vi "Upper Target Loop.vi"(11 "Camera Name":string="cam0") -> ()   [LabVIEW 2025]
uses:
  <vilib>/vision/NI_Vision_Development_Module.lvlib
  <vilib>/vision/Image Controls.llb/IMAQ Image.ctl
  <vilib>/Utility/config.llb/NI_LVConfig.lvlib
  <vilib>/Utility/config.llb/Write Key (String).vi
  Camera Set Up/Event/Event Setup Types.ctl
  <vilib>/Analysis/NI_AALBase.lvlib
  <vilib>/Analysis/baseanly.llb/Mean (DBL).vi
  <vilib>/Rock Robotics/Network Tables/NT Write Number.vi
  <vilib>/Utility/config.llb/Read Key (String).vi
  Camera Set Up/Ctrl/Camera Setup Cluster.ctl
panel:
  in  "Main":enum32{"Page 1", "Page 2"}(tab)
  in  "Settings":bool
  in  "Save":bool
  in  "Tools":bool
  out "Angle Array":dbl[](array[numeric]) format="%.1f"
  out "Distance  Array":dbl[](array[numeric]) format="%.1f"
  out "Avg Angle":dbl format="%0.2f"
  out "Avg Distance":dbl format="%0.2f"
  out "Image":T1(plugin-control)
  in  "Home":bool
  out "Mask":T1(plugin-control)
  in  "Dilate":bool
  in  "Color Range":T2={"Hue"={21.620689392089844, 69.62068939208984}, "Sat"={66.41378784179688, 255.0}, "Val"={96.0, 255.0}} {"Hue" scale=0.0..255.0 scale format="%#_3g"}
  in  "Height to center of target \n from floor (hp (in))":dbl=104.0 format="%#_13g"
  in  "FOV":dbl=120.0
  in  "Robot Calibration":T3={"Camera Height on robot (in)"=26.7, "Camera Angle on the robot (deg)"=21.6, "Slope"=0.946, "Offset"=10.775} {"Offset" format="%#_13g"; "Slope" format="%#_13g"; "Camera Angle on the robot (deg)" format="%#_13g"; "Camera Height on robot (in)" format="%#_13g"}
  in  "Score Threshold %":dbl=70.0
  in  "Size Limit %":dbl=0.02 format="%#_13g"
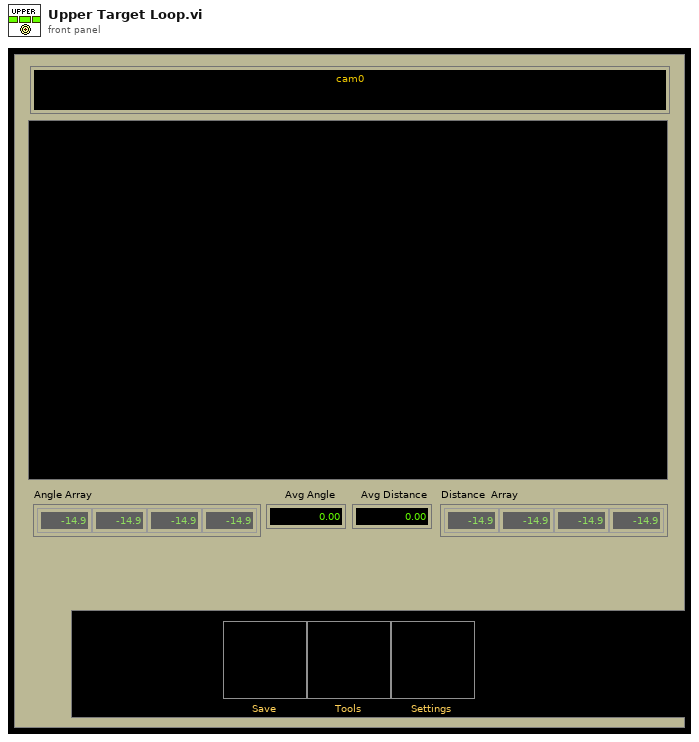
[diagram p1: front panel]
types:
  T1 = typedef "IMAQ Image.ctl" = refnum<image>
  T2 = cluster{"Hue":cluster{dbl, dbl}, "Sat":cluster{dbl, dbl}, "Val":cluster{dbl, dbl}}
  T3 = typedef "Camera Setup Cluster.ctl" = cluster{"Camera Height on robot (in)":dbl, "Camera Angle on the robot (deg)":dbl, "Slope":dbl, "Offset":dbl}
  T4 = typedef "Image Type" = u32
  T5 = typedef "Particle Parameters" = i32
  T6 = enum32{"AutoM", "Close", "Dilate", "Erode", "Gradient", "Gradient out", "Gradient in", "Hit miss", "Open", "PClose", "POpen", "Thick", "Thin"}
  T7 = typedef "Event Setup Types.ctl" = enum16{"Default", "Camera Loop Started", "GreyScale", "Reset Camera Settings", "Reset Team Number", "Save Data", "Setting Changed", "Update Video Mode", "Video Mode Changed", "Exit"}
  T8 = typedef "Event Setup Types.ctl" = enum16{"Default", "Camera Loop Started", "Close Settings", "GreyScale", "Open Front Panel", "Reset Team Number", "Save Data", "Exit"}
  T9 = typedef "Target Fields.ctl" = cluster{"diameter points":cluster{"first point":cluster{"x":dbl, "y":dbl}, "projected point":cluster{"x":dbl, "y":dbl}}, "normalized center":cluster{"x":dbl, "y":dbl}, "Overall Score":dbl, "Area Score":dbl, "Moment Score":dbl, "Aspect Score":dbl, "Distance (ft)":dbl, "Upper Goal":bool}
  T10 = typedef "NI_LVConfig.lvlib/Config Data RefNum.ctl" = refnum<k1>
  T11 = cluster{cluster{"Lower":dbl, "Upper":dbl}, cluster{"Lower":dbl, "Upper":dbl}, cluster{"Lower":dbl, "Upper":dbl}}
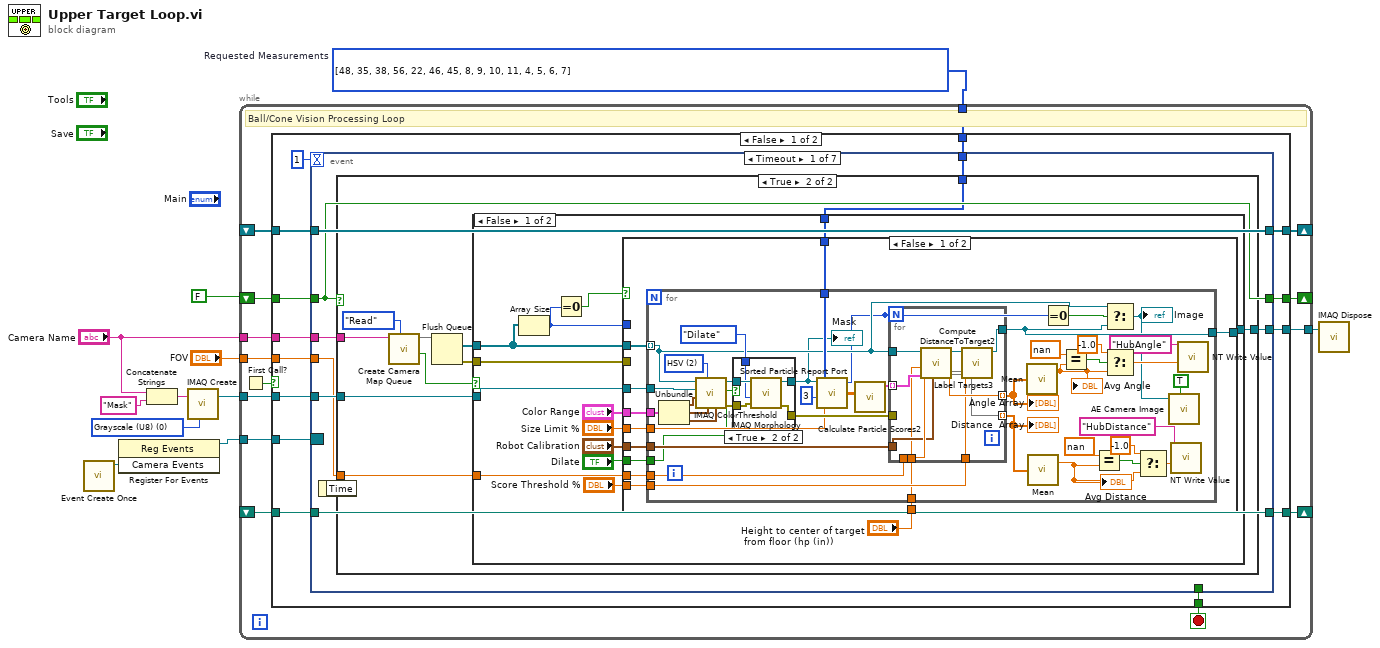
[diagram p0: block diagram]
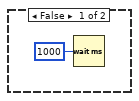
[diagram p2: hidden frame]
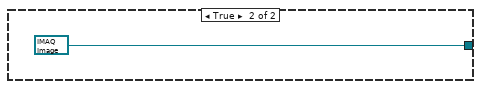
[diagram p4: hidden frame]
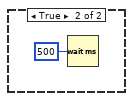
[diagram p5: hidden frame]
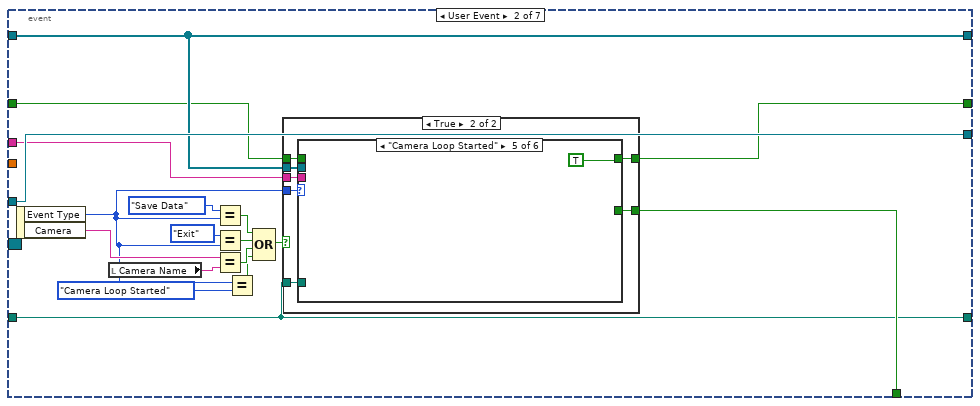
[diagram p6: hidden frame]
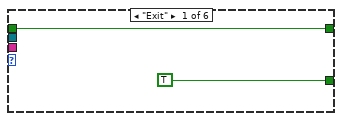
[diagram p8: hidden frame]
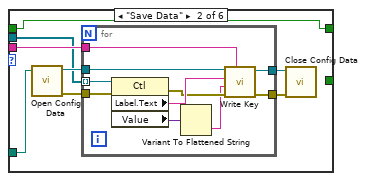
[diagram p9: hidden frame]
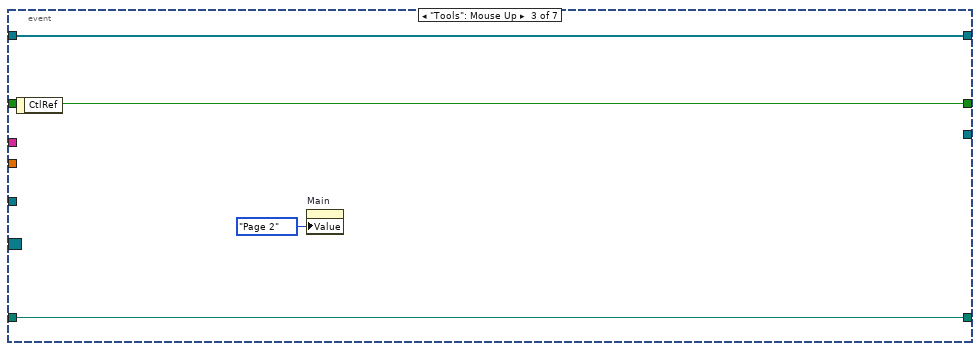
[diagram p13: hidden frame]
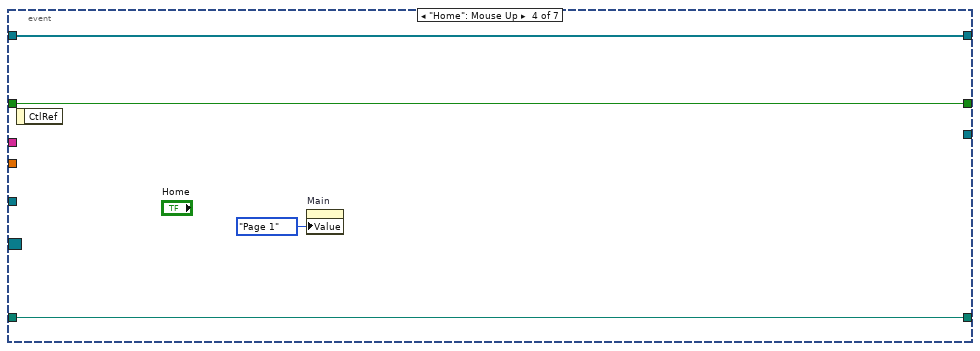
[diagram p14: hidden frame]
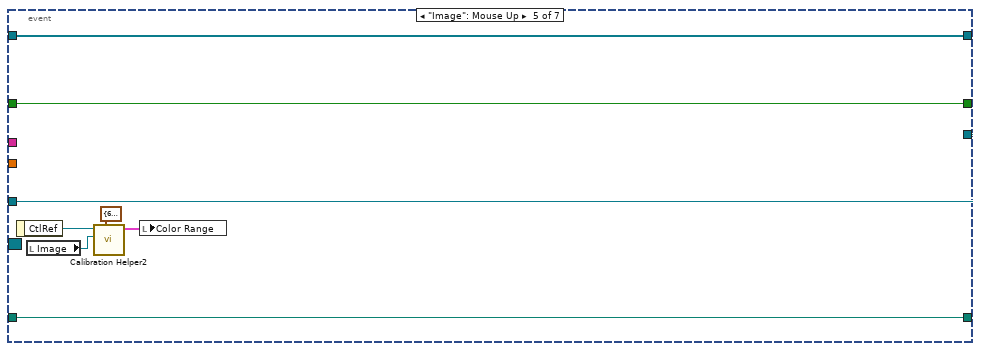
[diagram p15: hidden frame]
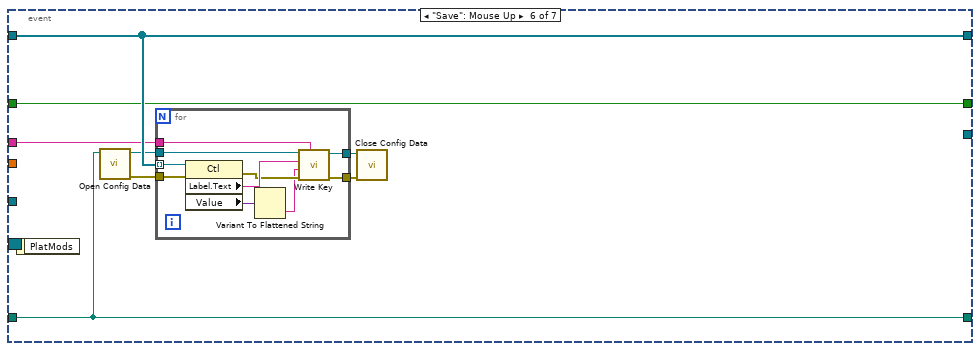
[diagram p16: hidden frame]
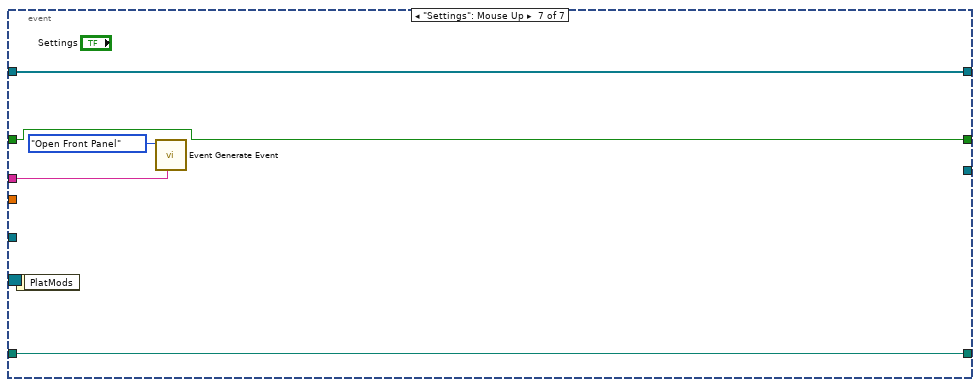
[diagram p17: hidden frame]
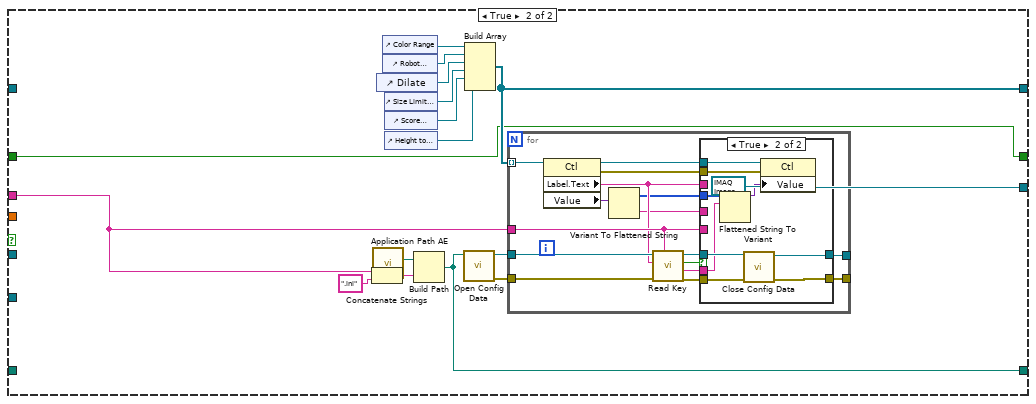
[diagram p18: hidden frame]
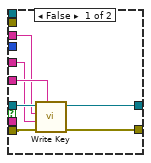
[diagram p19: hidden frame]
diagram:
  w7 = T4 0 items=["Grayscale (U8)", "Grayscale (I16)", "Grayscale (SGL)", "Complex (CSG)", "RGB (U32)", "HSL (U32)", "RGB (U64)", "Grayscale (U16)"] ("Image Type")
  w4 = T5[] [48, 35, 38, 56, 22, 46, 45, 8, 9, 10, 11, 4, 5, 6, 7] items=["Center of Mass X", "Center of Mass Y", "First Pixel X", "First Pixel Y", "Bounding Rect Left", "Bounding Rect Top", "Bounding Rect Right", "Bounding Rect Bottom", "Max Feret Diameter Start X", "Max Feret Diameter Start Y", "Max Feret Diameter End X", "Max Feret Diameter End Y", "Max Horiz. Segment Length Left", "Max Horiz. Segment Length Right", "Max Horiz. Segment Length Row", "-", "Bounding Rect Width", "Bounding Rect Height", "Bounding Rect Diagonal", "Perimeter", "Convex Hull Perimeter", "Holes' Perimeter", "Max Feret Diameter", "Equivalent Ellipse Major Axis", "Equivalent Ellipse Minor Axis", "Equivalent Ellipse Minor Axis (Feret)", "Equivalent Rect Long Side", "Equivalent Rect Short Side", "Equivalent Rect Diagonal", "Equivalent Rect Short Side (Feret)", "Average Horiz. Segment Length", "Average Vert. Segment Length", "Hydraulic Radius", "Waddel Disk Diameter", "-", "Area", "Holes' Area", "Particle & Holes' Area", "Convex Hull Area", "Image Area", "-", "Number of Holes", "Number of Horiz. Segments", "Number of Vert. Segments", "-", "Orientation", "Max Feret Diameter Orientation", "-", "% Area/Image Area", "% Area/(Particle & Holes' Area)", "Ratio of Equivalent Ellipse Axes", "Ratio of Equivalent Rect Sides", "-", "Elongation Factor", "Compactness Factor", "Heywood Circularity Factor", "Type Factor", "-", "Sum X", "Sum Y", "Sum XX", "Sum XY", "Sum YY", "Sum XXX", "Sum XXY", "Sum XYY", "Sum YYY", "-", "Moment of Inertia XX", "Moment of Inertia XY", "Moment of Inertia YY", "Moment of Inertia XXX", "Moment of Inertia XXY", "Moment of Inertia XYY", "Moment of Inertia YYY", "Norm. Moment of Inertia XX", "Norm. Moment of Inertia XY", "Norm. Moment of Inertia YY", "Norm. Moment of Inertia XXX", "Norm. Moment of Inertia XXY", "Norm. Moment of Inertia XYY", "Norm. Moment of Inertia YYY", "Hu Moment 1", "Hu Moment 2", "Hu Moment 3", "Hu Moment 4", "Hu Moment 5", "Hu Moment 6", "Hu Moment 7"]  # Requested Measurements
  n1 = call "Event Create Once.vi"() -> ("Camera Events"=w9:refnum<user-event>)  [unwired: 10 in, 1 out]
  n2 = register-events(w9) -> (reference out=w8:refnum<event-registration>)  [unwired: 2 in, 1 out]
  n3 = Concatenate Strings("Camera Name", "Mask" ("string")) -> (w6:string)
  n4 = call "IMAQ Create"("Image Name"=w6, "Image Type"=w7) -> ("New Image"=w11:T1)  [unwired: 2 in, 2 out]
  n5 = while {
    tunnel: w11 -> [w25]
    tunnel: w4 -> [w24]
    tunnel: [w23] -> w10
    tunnel: w8 -> [w22]
    tunnel: "FOV" -> [w20]
    tunnel: "Camera Name" -> [w19]
    shift-right: [w17] -> _
    shift-left: _ -> [w16]
    shift-right: [w15] -> _
    shift-left: _ -> [w14]
    shift-right: [w12] -> _
    shift-left: FALSE -> [w13]
    stop <- w21 stop-if-true
    # "Ball/Cone Vision Processing Loop"
    n6 = First Call?() -> (First Call?: T/F=w18:bool)
    n7 = case shown="False" w18 {
      tunnel: w25 -> [w39 _]
      tunnel: w24 -> [w38 _]
      tunnel: [w37 T1 refnum ("New Image")] -> w23
      tunnel: w22 -> [w35 _]
      tunnel: [w34 _] -> w21
      tunnel: w20 -> [w33 _]
      tunnel: w19 -> [w32 w245]
      tunnel: [w30 w244] -> w17
      tunnel: w16 -> [w31 _]
      tunnel: [w28 w243] -> w15
      tunnel: w14 -> [w29 _]
      tunnel: w13 -> [w27 w234]
      tunnel: [w26 w234] -> w12
      frame False {
        n8 = event shown="[0] Timeout" {
          selector: w35 -> [_ _ _ _ _ _ _]
          dyn-events: _ -> [_ _ _ _ _ _ _]
          timeout: 1 -> [_ _ _ _ _ _ _]
          tunnel: w39 -> [w45 w162 _ _ w208 _ _]
          tunnel: w38 -> [w43 _ _ _ _ _ _]
          tunnel: [w42 w162 _ _ w208 _ _] -> w37
          tunnel: [_ w161 _ _ _ _ _] -> w34
          tunnel: w33 -> [w44 _ _ _ _ _ _]
          tunnel: w32 -> [w41 w160 _ _ _ w216 w230]
          tunnel: w31 -> [w47 w158 w198 w202 w207 w217 w233]
          tunnel: [w47 w158 w198 w202 w207 w217 w233] -> w30
          tunnel: w29 -> [w46 w159 w197 w201 w206 w218 w232]
          tunnel: [w46 w159 w197 w201 w206 w218 w232] -> w28
          tunnel: [w40 w148 w195 w199 w203 w211 w229] -> w26
          tunnel: w27 -> [w40 w149 w195 w199 w203 w211 w229]
          event Timeout {
            n9 = event-data() -> ()  [unwired: 1 in, 1 out]
            n10 = case shown="True" w40 {
              tunnel: w45 -> [_ w57]
              tunnel: w44 -> [_ w56]
              tunnel: w43 -> [_ w55]
              tunnel: [_ w54] -> w42
              tunnel: w41 -> [_ w50]
              frame False {
                n11 = Wait (ms)(milliseconds to wait=u32 1000) -> ()  [unwired: 1 out]
              }
              frame True {
                n12 = call "Create Camera Map Queue.vi"("Action"=enum16{"Read", "Write"}."Read", "Camera"=w50) -> ("key not found?"=w49:bool, 3:w53)  [unwired: 7 in, 1 out]
                n13 = Flush Queue(queue=w53) -> (remaining elements=w51:T1[], error out=w52:errorcluster)  [unwired: 1 in, 1 out]
                n14 = case shown="False" w49 {
                  tunnel: w57 -> [w70 _]
                  tunnel: w56 -> [w69 _]
                  tunnel: w55 -> [w68 _]
                  tunnel: [w66 _] -> w54
                  tunnel: w52 -> [w65 _]
                  tunnel: w51 -> [w63 _]
                  frame False {
                    n15 = Array Size(array=w63) -> (size(s)=w60:i32)
                    n16 = Equal To 0?(x=w60) -> (x = 0?=w59:bool)
                    n17 = case shown="False" w59 {
                      tunnel: w68 -> [w83 _]
                      tunnel: w70 -> [w82 _]
                      tunnel: [w77 T1 refnum ("Image out")] -> w66
                      tunnel: "Color Range" -> [w81 _]
                      tunnel: "Size Limit %" -> [w80 _]
                      tunnel: "Robot Calibration" -> [w79 _]
                      tunnel: w69 -> [w78 _]
                      tunnel: "Dilate" -> [w76 _]
                      tunnel: w63 -> [w75 _]
                      tunnel: w65 -> [_ _]
                      tunnel: "Score Threshold %" -> [w74 _]
                      tunnel: "Height to center of target \n from floor (hp (in))" -> [w73 _]
                      tunnel: w60 -> [_ _]
                      frame False {
                        n18 = for {
                          tunnel: w83 -> [w124]
                          tunnel: w82 -> [w120]
                          tunnel: [w116] -> w77
                          tunnel: w75 -> [w109] mode=indexing
                          tunnel: w81 -> [w108]
                          tunnel: w80 -> [w107]
                          tunnel: w79 -> [w106]
                          tunnel: w78 -> [w105]
                          tunnel: w76 -> [w103]
                          tunnel: w74 -> [w101]
                          tunnel: w73 -> [w96]
                          w114 = u16 2 items=["RGB", "HSL", "HSV", "HSI"] ("Color Mode")
                          n19 = Unbundle(w108) -> ("Hue"=w121:cluster{dbl, dbl}, "Sat"=w123:cluster{dbl, dbl}, "Val"=w122:cluster{dbl, dbl})
                          n20 = call "IMAQ ColorThreshold"("Blue or Luma or Val or Inten Range"=w122, "Green or Sat Range"=w123, "Color Mode"=w114, "Red or Hue Range"=w121, "Image Dst"=w120, "Image Src"=w109) -> ("error out"=w111:errorcluster, "Image Dst Out"=w113:T1)  [unwired: 4 in]
                          n21 = case shown="True" w103 {
                            tunnel: w113 -> [w126 w131]
                            tunnel: [w126 w130] -> w102
                            tunnel: T6."Dilate" ("Operation") -> [_ w129]
                            tunnel: w111 -> [w125 w128]
                            tunnel: [w125 w127] -> w110
                            frame False {
                            }
                            frame True {
                              n22 = call "IMAQ Morphology"("error in (no error)"=w128, "Operation"=w129, "Image Src"=w131) -> ("error out"=w127:errorcluster, "Image Dst Out"=w130:T1)  [unwired: 7 in]
                            }
                          }
                          "Mask" <- w102
                          n23 = call "Sorted Particle Report Port.vi"("Min Area Size %"=w107, "Particle Count Limit"=3 ("Particle Count"), "Pixel Measurements"=w124, "Image in"=w102) -> ("Sorted Data"=w118:dbl[][], "Particles"=w104:i32)  [unwired: 1 out]
                          n24 = call "Calculate Particle Scores2.vi"("Sorted Data"=w118) -> ("Scores"=w117:T9[])  [unwired: 10 in]
                          n25 = for {
                            N: w104 -> [_]
                            tunnel: w117 -> [w137] mode=indexing
                            tunnel: [w136] -> w97 mode=indexing
                            tunnel: w105 -> [w138]
                            tunnel: w106 -> [w135]
                            tunnel: w110 -> [_]
                            tunnel: w109 -> [w141]
                            tunnel: [w142] -> w116
                            tunnel: [w134] -> w100 mode=indexing
                            tunnel: w101 -> [w133]
                            tunnel: w96 -> [w132]
                            n26 = call "Compute DistanceToTarget2.vi"(6:w135, 8:w137, "Camera Type"=w132, "Line"=w138, "Image Src"=w141) -> (0:w139, "Distance (ft)"=w136:dbl, "Image Dst Out"=w140:T1, 4:w134)  [unwired: 3 in]
                            n27 = call "Label Targets3.vi"("Score Threshold"=w133, "results"=w139, "Image in"=w140) -> ("Image out"=w142:T1)  [unwired: 8 in]
                          }
                          "Angle Array" <- w97
                          "Distance  Array" <- w100
                          n28 = call-poly <vilib>:"Mean.vi"("X"=w97) -> ("mean"=w86:dbl)  [unwired: 1 out]
                          "Avg Angle" <- w86
                          n29 = call-poly <vilib>:"Mean.vi"("X"=w100) -> ("mean"=w92:dbl)  [unwired: 1 out]
                          "Avg Distance" <- w92
                          n30 = Equal To 0?(x=w104) -> (x = 0?=w115:bool)
                          n31 = Equal?(x=nan, y=w86) -> (x = y?=w89:bool)
                          n32 = Equal?(x=nan, y=w92) -> (x = y?=w94:bool)
                          n33 = Select(t=w109, s=w115, f=w116) -> (s? t:f=w85:T1)
                          "Image" <- w85
                          n34 = Select(t=-1.0, s=w89, f=w86) -> (s? t:f=w87:dbl)
                          n35 = Select(t=-1.0, s=w94, f=w92) -> (s? t:f=w91:dbl)
                          n36 = call "AE Camera Image.vi"("Update"=TRUE, "Goal Camera"=w85) -> ()  [unwired: 9 in, 1 out]
                          n37 = call-poly <vilib>:"NT Write Value.vi"("value"=w91, "name"="HubDistance" ("Name")) -> ()  [unwired: 9 in, 1 out]
                          n38 = call-poly <vilib>:"NT Write Value.vi"("value"=w87, "name"="HubAngle" ("Name")) -> ()  [unwired: 9 in, 1 out]
                        }
                      }
                      frame True {
                      }
                    }
                  }
                  frame True {
                    n39 = Wait (ms)(milliseconds to wait=u32 500) -> ()  [unwired: 1 out]
                  }
                }
              }
            }
          }
          event User Event {
            n40 = event-data() -> ("Event Type"=w146:T7, "Camera"=w153:string)  [unwired: 1 in]
            n41 = local read "Camera Name"() -> (w152:string)
            n42 = Equal?(x=Event_Setup_Types."Save Data", y=w146) -> (x = y?=w154:bool)
            n43 = Equal?(x=Event_Setup_Types."Exit", y=w146) -> (x = y?=w156:bool)
            n44 = Equal?(x=w153, y=w152) -> (x = y?=w151:bool)
            n45 = Equal?(x=w146, y=Event_Setup_Types."Camera Loop Started" ("x")) -> (x = y?=w145:bool)
            n46 = Compound Arithmetic op=OR(w154, w156, w151, w145) -> (w150:bool)
            n47 = case shown="True" w150 {
              tunnel: w146 -> [_ w170]
              tunnel: [_ w169] -> w161
              tunnel: w160 -> [_ w168]
              tunnel: w159 -> [_ w167]
              tunnel: w158 -> [_ w166]
              tunnel: w149 -> [w163 w165]
              tunnel: [w163 w164] -> w148
              frame False {
              }
              frame True {
                n48 = case shown="\"Camera Loop Started\"" w170 {
                  tunnel: [TRUE _ _ _ _ _] -> w169
                  tunnel: w168 -> [_ w176 _ _ _ _]
                  tunnel: w167 -> [_ w175 _ _ _ _]
                  tunnel: w166 -> [_ w174 _ _ _ _]
                  tunnel: w165 -> [w171 w173 w191 w192 _ w194]
                  tunnel: [w171 w173 w191 w192 TRUE w194] -> w164
                  frame "Exit" {
                  }
                  frame "Save Data" {
                    n49 = call <vilib>:"Open Config Data.vi"("configuration file path"=w175) -> ("error out"=w177:errorcluster, "refnum"=w180:T10)  [unwired: 8 in, 1 out]
                    n50 = for {
                      tunnel: w174 -> [w188] mode=indexing
                      tunnel: w180 -> [w190]
                      tunnel: w176 -> [w189]
                      tunnel: [w185] -> w179
                      tunnel: [w183] -> w178
                      tunnel: w177 -> [w182]
                      n51 = property class="Ctl"(reference=w188, error in=w182) -> (error out=w184:errorcluster, "Label.Text"=w187:string, "Value"=w186:variant)  [unwired: 1 out]
                      n52 = Variant To Flattened String(Variant=w186) -> (data string=w181:string)  [unwired: 1 out]
                      n53 = call-poly <vilib>:"Write Key.vi"("section"=w189, "error in (no error)"=w184, "value"=w181, "key"=w187, "refnum"=w190) -> ("error out"=w183:errorcluster, "refnum out"=w185:T10)  [unwired: 4 in, 1 out]
                    }
                    n54 = call <vilib>:"Close Config Data.vi"("error in (no error)"=w178, "refnum"=w179) -> ()  [unwired: 8 in, 2 out]
                  }
                  frame Default {
                  }
                  frame "Default" {
                  }
                  frame "Camera Loop Started" {
                  }
                  frame "Default" {
                  }
                }
              }
            }
          }
          event "Tools": Mouse Up {
            n55 = event-data() -> ()  [unwired: 1 in, 1 out]
            n56 = property on="Main" class="TabCtl (strict)"("Value"=enum32{"Page 1", "Page 2"}."Page 2" ("Main")) -> ()  [unwired: 2 in, 2 out]
          }
          event "Home": Mouse Up {
            n57 = event-data() -> ()  [unwired: 1 in, 1 out]
            n58 = property on="Main" class="TabCtl (strict)"("Value"=enum32{"Page 1", "Page 2"}."Page 1" ("Main")) -> ()  [unwired: 2 in, 2 out]
          }
          event "Image": Mouse Up {
            n59 = event-data() -> ("CtlRef"=w205:refnum<vi>)  [unwired: 1 in]
            n60 = local read "Image"() -> (w204:T1)
            n61 = call "Calibration Helper2.vi"("Std Devs"=cluster{"H":dbl, "S":dbl, "V":dbl} {"H"=6.0, "S"=6.0, "V"=6.0} ("Std Devs Ball"), "Image"=w204, "Image Ctl Refnum"=w205) -> ("output color"=w209:T11)  [unwired: 7 in, 1 out]
            n62 = local write "Color Range"(w209) -> ()
          }
          event "Save": Mouse Up {
            n63 = event-data() -> ()  [unwired: 1 in, 1 out]
            n64 = call <vilib>:"Open Config Data.vi"("configuration file path"=w218) -> ("error out"=w212:errorcluster, "refnum"=w215:T10)  [unwired: 8 in, 1 out]
            n65 = for {
              tunnel: w217 -> [w226] mode=indexing
              tunnel: w215 -> [w228]
              tunnel: w216 -> [w227]
              tunnel: [w223] -> w214
              tunnel: [w221] -> w213
              tunnel: w212 -> [w220]
              n66 = property class="Ctl"(reference=w226, error in=w220) -> (error out=w222:errorcluster, "Label.Text"=w225:string, "Value"=w224:variant)  [unwired: 1 out]
              n67 = Variant To Flattened String(Variant=w224) -> (data string=w219:string)  [unwired: 1 out]
              n68 = call-poly <vilib>:"Write Key.vi"("section"=w227, "error in (no error)"=w222, "value"=w219, "key"=w225, "refnum"=w228) -> ("error out"=w221:errorcluster, "refnum out"=w223:T10)  [unwired: 4 in, 1 out]
            }
            n69 = call <vilib>:"Close Config Data.vi"("error in (no error)"=w213, "refnum"=w214) -> ()  [unwired: 8 in, 2 out]
          }
          event "Settings": Mouse Up {
            n70 = event-data() -> ()  [unwired: 1 in, 1 out]
            n71 = call "Event Generate Event.vi"("Camera Name"=w230, "Event Type"=Event_Setup_Types."Open Front Panel") -> ()  [unwired: 10 in]
          }
        }
      }
      frame True {
        n72 = Concatenate Strings(w245, ".ini" ("name or relative path")) -> (w250:string)
        n73 = call "Application Path AE.vi"() -> ("Application Path out"=w238:path)  [unwired: 11 in]
        n74 = control-ref of="Dilate"() -> (w239:refnum<vi>)
        n75 = control-ref of="Color Range"() -> (w241:refnum<vi>)
        n76 = control-ref of="Robot Calibration"() -> (w240:refnum<vi>)
        n77 = control-ref of="Size Limit %"() -> (w237:refnum<vi>)
        n78 = control-ref of="Score Threshold %"() -> (w236:refnum<vi>)
        n79 = control-ref of="Height to center of target \n from floor (hp (in))"() -> (w235:refnum<vi>)
        n80 = Build Path(base path=w238, name or relative path=w250) -> (appended path=w243:path)
        n81 = call <vilib>:"Open Config Data.vi"("configuration file path"=w243) -> ("error out"=w242:errorcluster, "refnum"=w249:T10)  [unwired: 8 in, 1 out]
        n82 = Build Array(w241, w240, w239, w237, w236, w235) -> (w244:refnum<vi>[])
        n83 = for {
          tunnel: w249 -> [w267]
          tunnel: w245 -> [w260]
          tunnel: w244 -> [w266] mode=indexing
          tunnel: [w258] -> w248
          tunnel: [w256] -> w247
          tunnel: w242 -> [w252]
          n84 = property class="Ctl"(reference=w266) -> (reference out=w263:refnum<vi>, error out=w262:errorcluster, "Label.Text"=w259:string, "Value"=w255:variant)  [unwired: 1 in]
          n85 = Variant To Flattened String(Variant=w255) -> (data string=w254:string, 1:w253:i16[])
          n86 = call-poly <vilib>:"Read Key.vi"("section"=w260, "error in (no error)"=w252, "key"=w259, "refnum"=w267) -> ("error out"=w257:errorcluster, "value"=w264:string, "found?"=w265:bool, "refnum out"=w261:T10)  [unwired: 4 in]
          n87 = case shown="True" w265 {
            tunnel: w264 -> [_ w276]
            tunnel: w263 -> [_ w281]
            tunnel: w262 -> [_ w280]
            tunnel: w261 -> [w274 w279]
            tunnel: w260 -> [w273 _]
            tunnel: w259 -> [w272 _]
            tunnel: [w271 w279] -> w258
            tunnel: w257 -> [w270 w278]
            tunnel: [w269 w278] -> w256
            tunnel: w254 -> [w268 _]
            tunnel: w253 -> [_ w277]
            frame False {
              n88 = call-poly <vilib>:"Write Key.vi"("section"=w273, "error in (no error)"=w270, "value"=w268, "key"=w272, "refnum"=w274) -> ("error out"=w269:errorcluster, "refnum out"=w271:T10)  [unwired: 4 in, 1 out]
            }
            frame True {
              n89 = Flattened String To Variant(6:w276, 7:w277) -> (3:w275:variant)  [unwired: 1 in, 1 out]
              n90 = property class="Ctl"(reference=w281, error in=w280, "Value"=w275) -> ()  [unwired: 2 out]
            }
          }
        }
        n91 = call <vilib>:"Close Config Data.vi"("error in (no error)"=w247, "refnum"=w248) -> ()  [unwired: 8 in, 2 out]
      }
    }
  }
  n92 = call "IMAQ Dispose"("Image"=w10) -> ()  [unwired: 5 in, 1 out]
